vi "SDPORTUPDT.vi"(8 "error in (no error)":errorcluster, 10 "Command":string, 11 "UI Actor in":refnum<class "UI Actor.lvclass">) -> (0 "error out":errorcluster)   [LabVIEW 2020, in "UI Actor.lvlib" / "UI Actor.lvclass"]
uses:
  UI Actor.lvclass
  UI Actor.lvclass/UI Actor.ctl
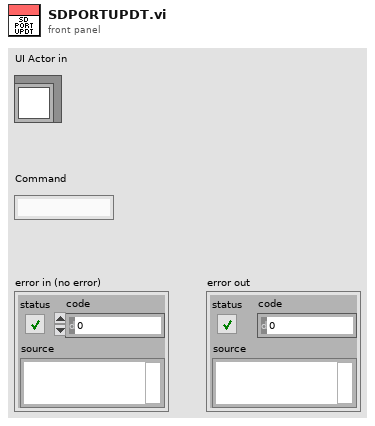
[diagram p1: front panel]
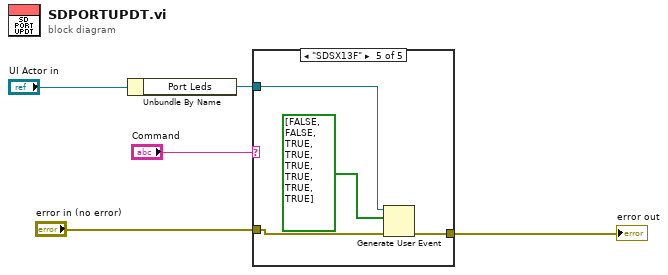
[diagram p0: block diagram]
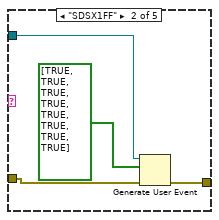
[diagram p3: hidden frame]
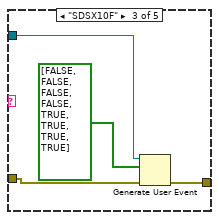
[diagram p4: hidden frame]
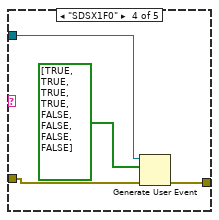
[diagram p5: hidden frame]
diagram:
  n1 = Unbundle By Name("UI Actor in") -> ("Port Leds"=w2:refnum<user-event>)
  n2 = case shown="\"SDSX13F\"" "Command" {
    tunnel: [_ w9 w13 w17 w21] -> w5
    tunnel: "error in (no error)" -> [_ w8 w12 w16 w20]
    tunnel: w2 -> [_ w7 w11 w15 w19]
    frame "False", Default {
    }
    frame "SDSX1FF" {
      n3 = Generate User Event(user event=w7, event data cluster=bool[] [TRUE, TRUE, TRUE, TRUE, TRUE, TRUE, TRUE, TRUE] ("event data"), error in=w8) -> (error out=w9:errorcluster)  [unwired: 1 in, 1 out]
    }
    frame "SDSX10F" {
      n4 = Generate User Event(user event=w11, event data cluster=bool[] [FALSE, FALSE, FALSE, FALSE, TRUE, TRUE, TRUE, TRUE] ("event data"), error in=w12) -> (error out=w13:errorcluster)  [unwired: 1 in, 1 out]
    }
    frame "SDSX1F0" {
      n5 = Generate User Event(user event=w15, event data cluster=bool[] [TRUE, TRUE, TRUE, TRUE, FALSE, FALSE, FALSE, FALSE] ("event data"), error in=w16) -> (error out=w17:errorcluster)  [unwired: 1 in, 1 out]
    }
    frame "SDSX13F" {
      n6 = Generate User Event(user event=w19, event data cluster=bool[] [FALSE, FALSE, TRUE, TRUE, TRUE, TRUE, TRUE, TRUE] ("event data"), error in=w20) -> (error out=w21:errorcluster)  [unwired: 1 in, 1 out]
    }
  }
  "error out" <- w5
